vi "SIMA.vi"(8 "error in":errorcluster, 9 "tsh":dbl, 10 "focus":dbl, 11 "In":T1) -> (0 "error out":errorcluster, 1 "Out":T1, 2 "Intensity fit gausian for SM":dbl[][](graph), 3 "Coefficiens":dbl[][](array[numeric]), 7 "Intensity for ft debug color":dbl[][](graph))   [LabVIEW 2009]
uses:
  <vilib>/vision/Image Controls.llb/IMAQ Image.ctl
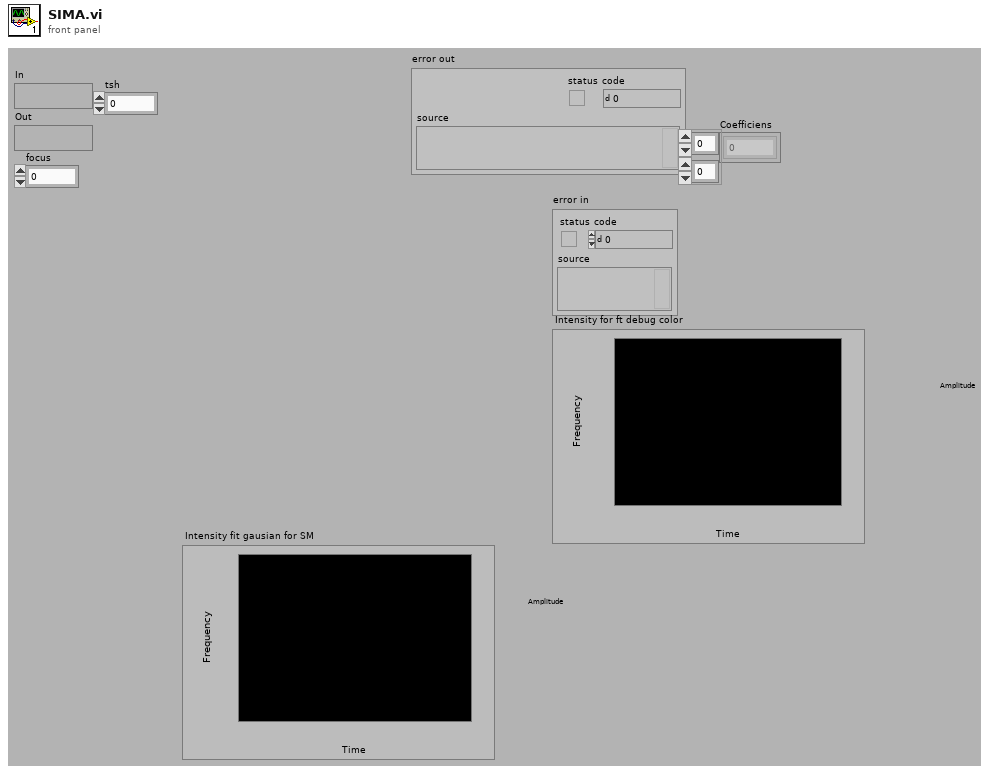
[diagram p1: front panel]
types:
  T1 = typedef "IMAQ Image.ctl" = refnum<image>
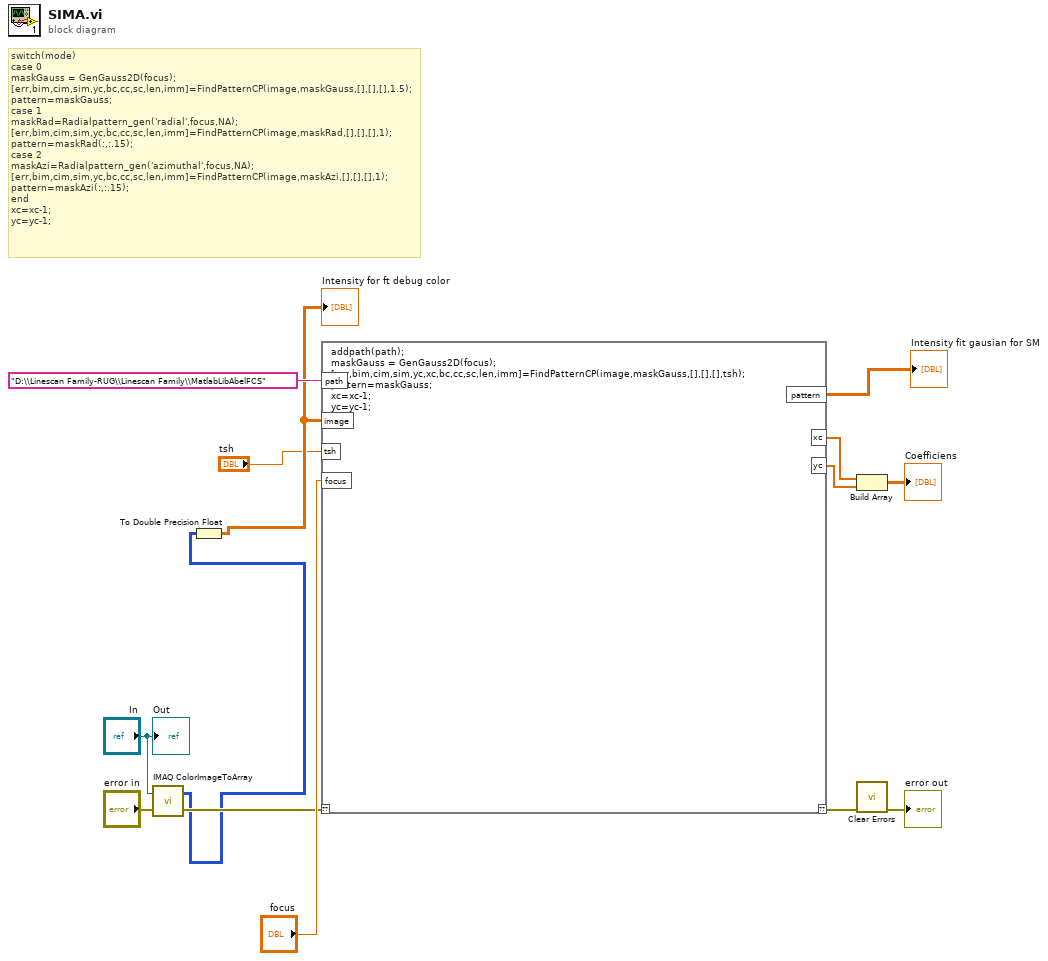
[diagram p0: block diagram]
diagram:
  # "switch(mode)\ncase 0\nmaskGauss = GenGauss2D(focus);\n[err,bim,cim,sim,yc,bc,cc,sc,len,imm]=FindPatternCP(image,maskGauss,[],[],[],1.5);\npattern=maskGauss;\ncase 1\nmaskRad=Radialpattern_gen('radial',focus,NA);\n[err,bim,cim,sim,yc,bc,cc,sc,len,imm]=FindPatternCP(image,maskRad,[],[],[],1);\npattern=maskRad(:,:.15);\ncase 2\nmaskAzi=Radialpattern_gen('azimuthal',focus,NA);\n[err,bim,cim,sim,yc,bc,cc,sc,len,imm]=FindPatternCP(image,maskAzi,[],[],[],1);\npattern=maskAzi(:,:.15);\nend\nxc=xc-1;\nyc=yc-1;"
  n1 = call "IMAQ ColorImageToArray"("Image"="In", "error in (no error)"="error in") -> ("Image Pixels (U32)"=w3:u32[][], "error out"=w10:errorcluster)  [unwired: 2 in, 1 out]
  n2 = To Double Precision Float(number=w3) -> (double precision float=w2:dbl[][])
  "Intensity for ft debug color" <- w2
  n3 = script code="addpath(path);\nmaskGauss = GenGauss2D(focus);\n[err,bim,cim,sim,yc,xc,bc,cc,sc,len,imm]=FindPatternCP(image,maskGauss,[],[],[],tsh);\npattern=maskGauss;\nxc=xc-1;\nyc=yc-1;"("??"=w10, "image"=w2, "path"="D:\\Linescan Family-RUG\\Linescan Family\\MatlabLibAbelFCS", "focus"="focus", "tsh"="tsh") -> ("??"=w12:errorcluster, "pattern"=→"Intensity fit gausian for SM":dbl[][], "xc"=w7:dbl[], "yc"=w6:dbl[])
  n4 = Build Array(w7, w6) -> (→"Coefficiens":dbl[][])
  n5 = call <vilib>:"Clear Errors.vi"("error in (no error)"=w12) -> ("error out"=→"error out":errorcluster)  [unwired: 6 in]
  "Out" <- "In"
